vi "Camera Config_Luan2024.05.01.vi"(6 "Extended shutter":bool=TRUE, 8 "error in (no error)":errorcluster, 9 "Exposure Time":dbl, 10 "Gain":dbl, 11 "IMAQDx session In":T1) -> (0 "error out":errorcluster, 3 "IMAQDx session Out":T1)   [LabVIEW 2023]
uses:
  <vilib>/userDefined/High Color/IMAQdx.ctl
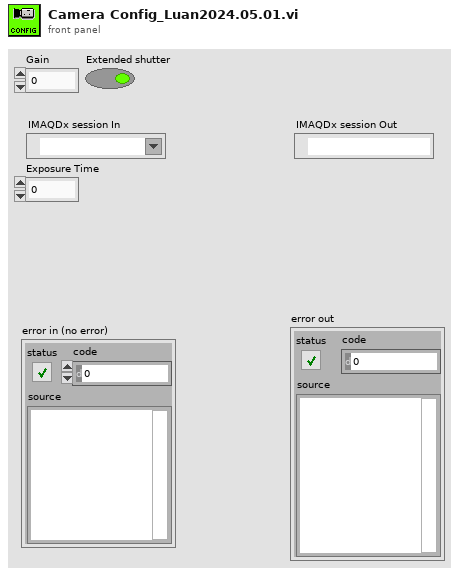
[diagram p1: front panel]
types:
  T1 = typedef "IMAQdx.ctl" = refnum<k21>
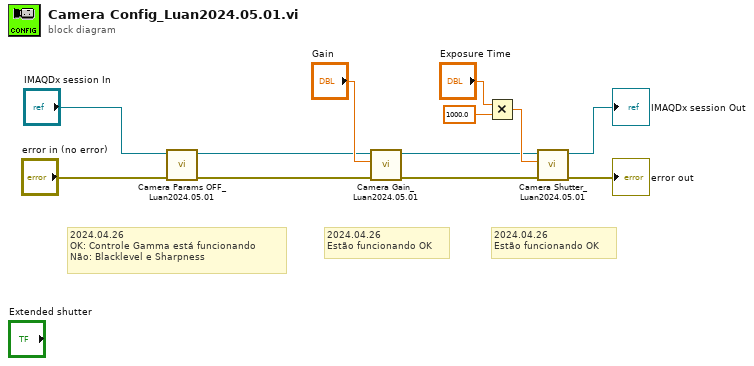
[diagram p0: block diagram]
diagram:
  # "2024.04.26\nOK: Controle Gamma está funcionando\nNão: Blacklevel e Sharpness"
  # "2024.04.26\nEstão funcionando OK"
  # "2024.04.26\nEstão funcionando OK"
  n1 = call "Camera Params OFF_Luan2024.05.01.vi"("error in (no error)"="error in (no error)", "IMAQDx session In"="IMAQDx session In") -> ("error out"=w3:errorcluster, "IMAQDx session out"=w4:T1)  [unwired: 8 in]
  n2 = call "Camera Gain_Luan2024.05.01.vi"("error in (no error)"=w3, "x"="Gain", "Refnum in"=w4) -> ("error out"=w6:errorcluster, "Refnum out"=w7:T1)  [unwired: 6 in, 1 out]
  n3 = Multiply(x="Exposure Time", y=1000.0) -> (x*y=w10:dbl)
  n4 = call "Camera Shutter_Luan2024.05.01.vi"("error in (no error)"=w6, "Exposure Time"=w10, "Refnum in"=w7) -> ("error out"=→"error out":errorcluster, "Refnum out"=→"IMAQDx session Out":T1)  [unwired: 7 in]
